vi "Main.vi"(0 "This Module":T1, 11 "error in (no error)":errorcluster) -> (15 "error out":errorcluster)   [LabVIEW 2017, in "Template.lvlib"]
doc: "This VI is the Module VI containing all the code required from this Module"
uses:
  Template.lvlib
  Modules.ctl
  Controls/Module - Data.ctl
  Controls/Module - States.ctl
  Controls/Timing - Data.ctl
  Controls/Process - Element.ctl
  Controls/Process.ctl
  Controls/Process - Status.ctl
  Controls/Timing - Mode.ctl
  Controls/Message - Queue Manager Mode.ctl
  Error Handler - Logger Module/Controls/Message.ctl
  Error Handler - Logger Module/Controls/Module - States.ctl
  Controls/FP - Update Value.ctl
  Controls/FP - Actionable Element.ctl
  Controls/FP - Enable_Disable.ctl
  Controls/Timing - Setup.ctl
  Error Handler - Logger Module/Error Handler - Logger.lvlib
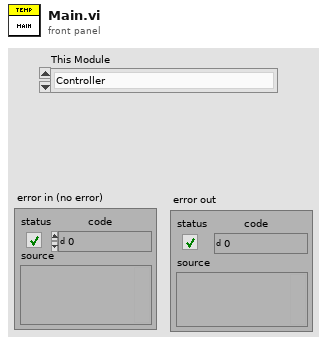
[diagram p1: front panel]
types:
  T1 = typedef "Error Handler - Logger.lvlib/Modules.ctl" = enum16{"Controller", "Error Handler - Logger"}
  T2 = typedef "Template.lvlib/Message - Queue Manager Mode.ctl" = enum16{"Create", "Get", "Destroy"}
  T3 = typedef "Template.lvlib/Timing - Mode.ctl" = enum16{"Reset", "Read", "Pause", "Resume"}
  T4 = typedef "Template.lvlib/Module - Data.ctl" = cluster{"This Module":T1, "Current State":T5, "Timing Data":T6, "Processes":T7[], "Log":string}
  T5 = typedef "Template.lvlib/Module - States.ctl" = enum16{"Initialize", "Event ", "Send data", "FP Element: Update", "FP Element: Disable/Enable", "Timer: Setup", "Terminate", "---------------Template---------------"}
  T6 = typedef "Template.lvlib/Timing - Data.ctl" = cluster{"Elapsed Time":dbl, "Time Target":dbl, "Time Stamp":timestamp, "Paused?":bool, "Reached?":bool}
  T7 = typedef "Template.lvlib/Process - Element.ctl" = cluster{"Process":T8, "Status":T9, "Data":variant}
  T8 = typedef "Template.lvlib/Process.ctl" = enum16{""}
  T9 = typedef "Template.lvlib/Process - Status.ctl" = enum16{"Uninitialized", "Busy"}
  T10 = typedef "Error Handler - Logger.lvlib/Message.ctl" = cluster{"State":T11, "Data":variant, "Originating Module":T1}
  T11 = typedef "Error Handler - Logger.lvlib/Module - States.ctl" = enum16{"Initialize", "Event ", "Send data", "FP Element: Update", "FP Element: Disable/Enable", "Timer: Setup", "Terminate", "--------Template----------", "Process Error", "Log ", "Log Error"}
  T12 = typedef "Template.lvlib/FP - Update Value.ctl" = cluster{"FP Element":T13, "Value":string}
  T13 = typedef "Template.lvlib/FP - Actionable Element.ctl" = enum16{"Put here all controls and indicators", "belonging to the UI of this module", "whose value can ", "be updated programatically", "or which can be enabled or disabled", ""}
  T14 = typedef "Template.lvlib/FP - Enable_Disable.ctl" = cluster{"FP Element":T13, "Enable?":bool}
  T15 = typedef "Template.lvlib/Timing - Setup.ctl" = cluster{"Mode":T3, "Update Time Target?":bool, "Time Target":dbl}
  T16 = typedef "Template.lvlib/Message.ctl" = cluster{"State":T5, "Data":variant, "Transitioning State?":bool}
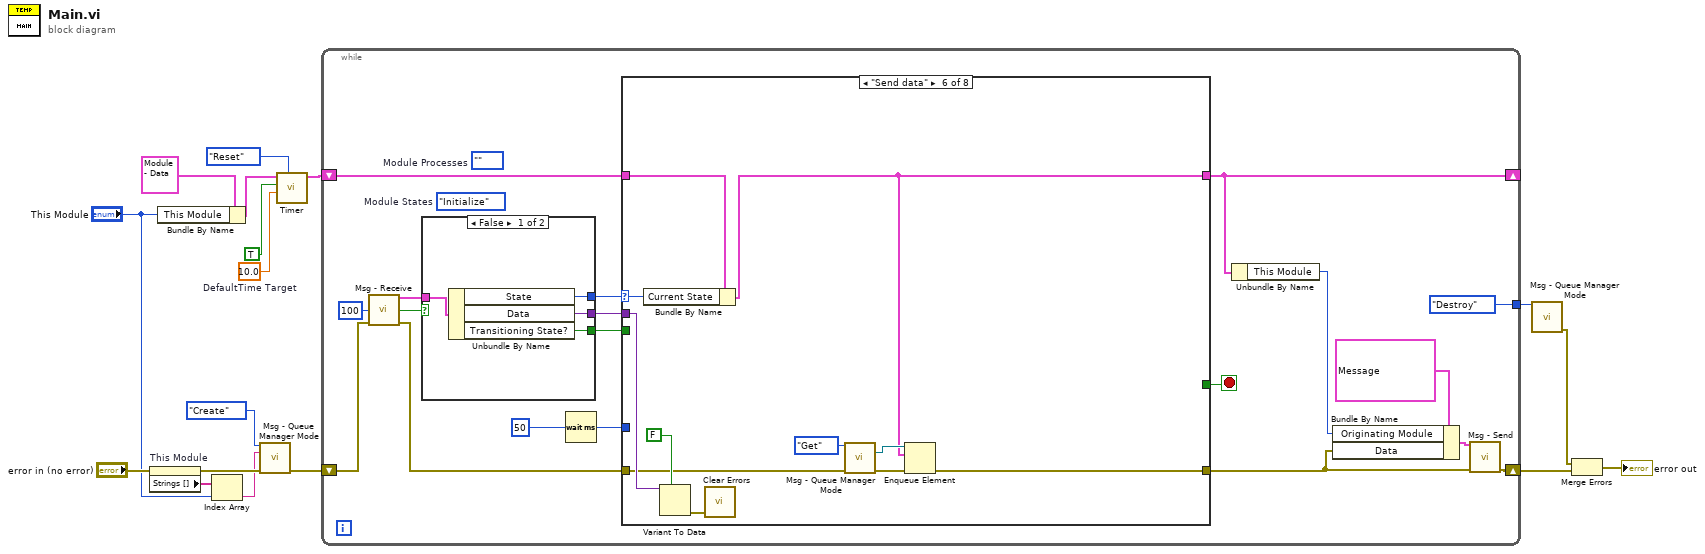
[diagram p0: block diagram]
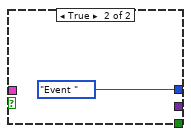
[diagram p2: hidden frame]
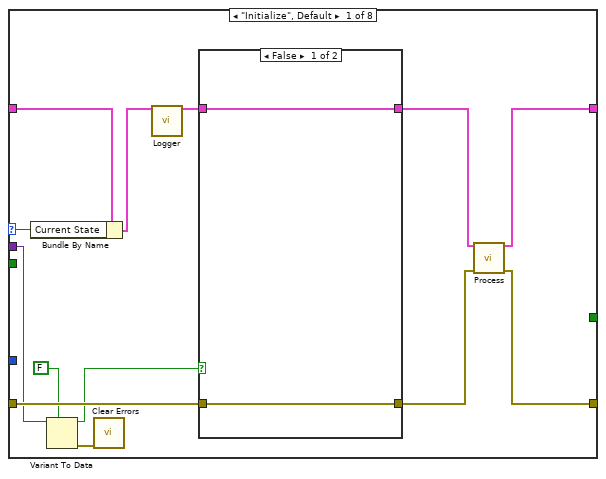
[diagram p3: hidden frame]
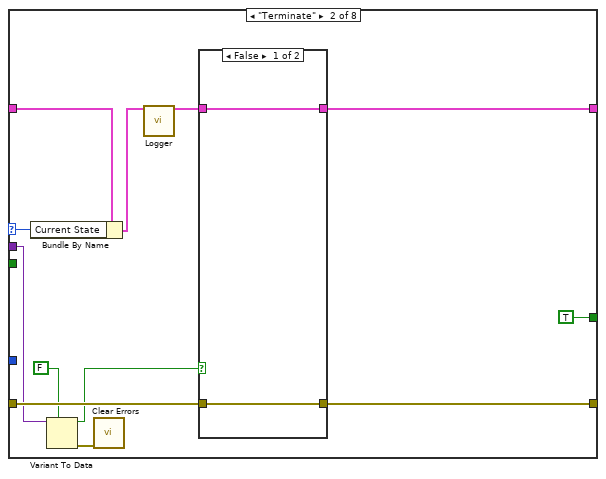
[diagram p5: hidden frame]
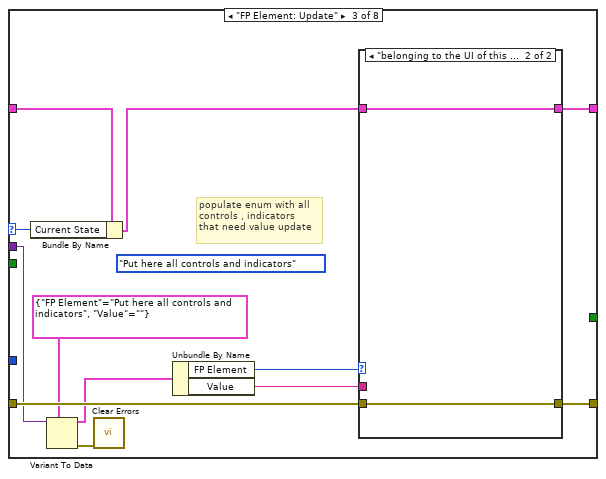
[diagram p7: hidden frame]
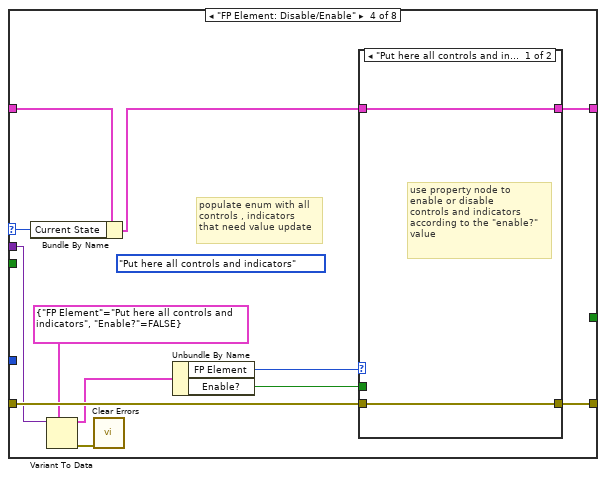
[diagram p9: hidden frame]
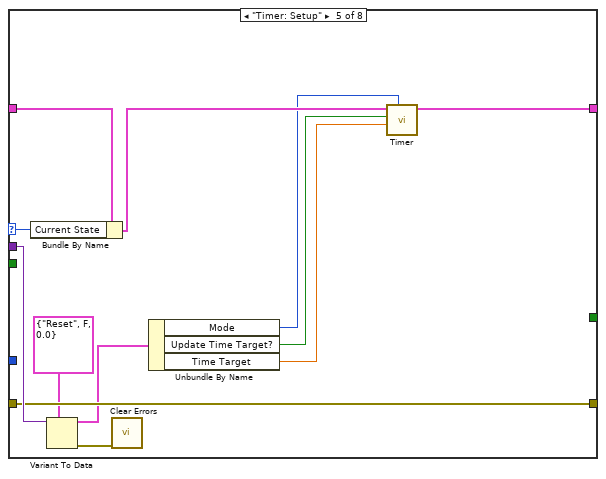
[diagram p11: hidden frame]
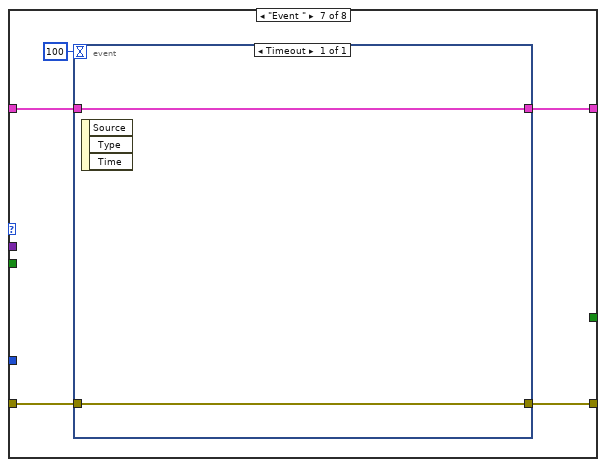
[diagram p12: hidden frame]
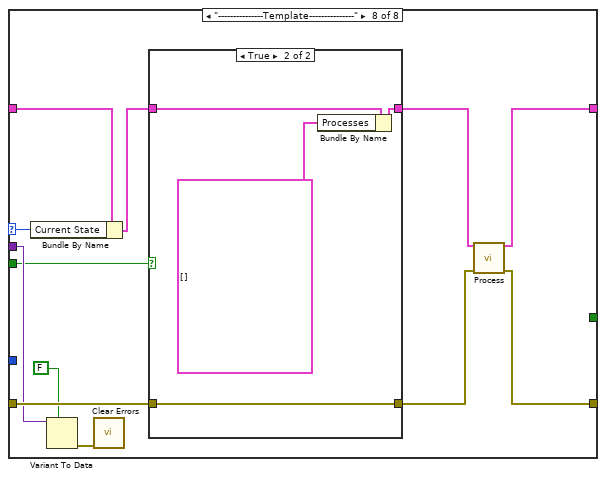
[diagram p13: hidden frame]
diagram:
  w13 = 10.0  # DefaultTime Target
  n1 = property on="This Module" class="Enum (strict)"(error in="error in (no error)") -> (error out=w8:errorcluster, "Strings []"=w10:string[])  [unwired: 1 in, 1 out]
  n2 = Bundle By Name(cluster=T4 {"This Module"=enum."Controller", "Current State"=enum."Initialize", "Timing Data"={"Elapsed Time"=0.0, "Time Target"=0.0, "Time Stamp"=timestamp(0 s since 1904-01-01), "Paused?"=FALSE, "Reached?"=FALSE}, "Processes"=[], "Log"=""} ("Module Data In"), "This Module"="This Module") -> (w16:T4)
  n3 = Index Array(array=w10, index="This Module") -> (element=w7:string)
  n4 = call "Msg - Queue Manager Mode.vi"("Mode"=Message_-_Queue_Manager_Mode."Create", "Module Name"=w7, "error in (no error)"=w8) -> ("error out"=w6:errorcluster)  [unwired: 10 in, 2 out]
  n5 = call "Timer.vi"("Mode"=Timing_-_Mode."Reset", "Time Target"=w13, "Update Target?"=TRUE, "Module Data In"=w16) -> ("Module Data Out"=w15:T4)  [unwired: 4 in, 3 out]
  n6 = while {
    shift-right: [w24] -> _
    shift-left: w15 -> [w36]
    shift-right: [w23] -> w3
    shift-left: w6 -> [w34]
    tunnel: [Message_-_Queue_Manager_Mode."Destroy" ("Mode")] -> w1
    stop <- w25 stop-if-true
    (unwired) Process.""  # Module Processes
    (unwired) Module_-_States."Initialize"  # Module States
    n7 = call "Msg - Receive.vi"("Timeout (ms)"=100, "error in (no error)"=w34) -> ("Message"=w30:T16, "timed out?"=w31:bool, "error out"=w33:errorcluster)  [unwired: 11 in]
    n8 = case shown="False" w31 {
      tunnel: w30 -> [w40 _]
      tunnel: [w39 Module_-_States."Event " ("State")] -> w29
      tunnel: [w38 _] -> w28
      tunnel: [w37 _] -> w19
      frame False {
        n9 = Unbundle By Name(w40) -> ("State"=w39:T5, "Data"=w38:variant, "Transitioning State?"=w37:bool)
      }
      frame True {
      }
    }
    n10 = Wait (ms)(milliseconds to wait=u32 50) -> (millisecond timer value=w26:u32)
    n11 = case shown="\"Send data\"" w29 {
      selector: w29 -> [w54 w70 w86 w102 w118 w129 _ w148]
      tunnel: [w48 w64 w81 w97 w110 w124 w131 w142] -> w24
      tunnel: w36 -> [w53 w69 w85 w101 w117 w128 w132 w147]
      tunnel: [w45 w63 w80 w96 w115 w122 w133 w139] -> w18
      tunnel: w33 -> [w52 w68 w83 w99 w115 w123 w134 w145]
      tunnel: w28 -> [w51 w67 w82 w98 w116 w127 _ w144]
      tunnel: w26 -> [_ _ _ _ _ _ _ _]
      tunnel: [_ TRUE _ _ _ _ _ _] -> w25
      tunnel: w19 -> [_ _ _ _ _ _ _ w137]
      frame "Initialize", Default {
        n12 = Bundle By Name(cluster=w53, "Current State"=w54) -> (w43:T4)
        n13 = Variant To Data(type=FALSE, Variant=w51) -> (data=w49:bool, error out=w44:errorcluster)  [unwired: 1 in]
        n14 = call <vilib>:"Clear Errors.vi"("error in (no error)"=w44) -> ()  [unwired: 5 in, 2 out]
        n15 = call "Logger.vi"("Module Data In"=w43) -> ("Module Data Out"=w42:T4)  [unwired: 13 in, 1 out]
        n16 = case shown="False" w49 {
          tunnel: w42 -> [w56 w58]
          tunnel: [w56 w58] -> w47
          tunnel: w52 -> [w55 w57]
          tunnel: [w55 w57] -> w46
          frame False {
          }
          frame True {
          }
        }
        n17 = call "Process.vi"("Module Data In"=w47, "error in (no error)"=w46) -> ("Module Data Out"=w48:T4, "error out"=w45:errorcluster)  [unwired: 12 in]
      }
      frame "Terminate" {
        n18 = Bundle By Name(cluster=w69, "Current State"=w70) -> (w60:T4)
        n19 = Variant To Data(type=FALSE, Variant=w67) -> (data=w65:bool, error out=w62:errorcluster)  [unwired: 1 in]
        n20 = call <vilib>:"Clear Errors.vi"("error in (no error)"=w62) -> ()  [unwired: 5 in, 2 out]
        n21 = call "Logger.vi"("Module Data In"=w60) -> ("Module Data Out"=w59:T4)  [unwired: 13 in, 1 out]
        n22 = case shown="False" w65 {
          tunnel: w59 -> [w72 w74]
          tunnel: [w72 w74] -> w64
          tunnel: w68 -> [w71 w73]
          tunnel: [w71 w73] -> w63
          frame False {
          }
          frame True {
          }
        }
      }
      frame "FP Element: Update" {
        (unwired) FP_-_Actionable_Element."Put here all controls and indicators" ("FP Element")
        # "populate enum with all\ncontrols , indicators \nthat need value update"
        n23 = Bundle By Name(cluster=w85, "Current State"=w86) -> (w84:T4)
        n24 = Variant To Data(type=T12 {"FP Element"=enum."Put here all controls and indicators", "Value"=""} ("Message"), Variant=w82) -> (data=w77:T12, error out=w79:errorcluster)  [unwired: 1 in]
        n25 = call <vilib>:"Clear Errors.vi"("error in (no error)"=w79) -> ()  [unwired: 5 in, 2 out]
        n26 = Unbundle By Name(w77) -> ("FP Element"=w76:T13, "Value"=w75:string)
        n27 = case shown="\"belonging to the UI of this module\"" w76 {
          tunnel: w84 -> [w88 w90]
          tunnel: [w88 w90] -> w81
          tunnel: w83 -> [w87 w89]
          tunnel: [w87 w89] -> w80
          tunnel: w75 -> [_ _]
          frame "Put here all controls and indicators", Default {
            # "use property node to\nupdate the values of\ncorresponding\ncontrols and indicators"
          }
          frame "belonging to the UI of this module" {
          }
        }
      }
      frame "FP Element: Disable/Enable" {
        (unwired) FP_-_Actionable_Element."Put here all controls and indicators" ("FP Element")
        # "populate enum with all\ncontrols , indicators \nthat need value update"
        n28 = Bundle By Name(cluster=w101, "Current State"=w102) -> (w100:T4)
        n29 = Variant To Data(type=T14 {"FP Element"=enum."Put here all controls and indicators", "Enable?"=FALSE} ("Message"), Variant=w98) -> (data=w94:T14, error out=w95:errorcluster)  [unwired: 1 in]
        n30 = call <vilib>:"Clear Errors.vi"("error in (no error)"=w95) -> ()  [unwired: 5 in, 2 out]
        n31 = Unbundle By Name(w94) -> ("FP Element"=w93:T13, "Enable?"=w92:bool)
        n32 = case shown="\"Put here all controls and indicators\", Default" w93 {
          tunnel: w100 -> [w104 w106]
          tunnel: [w104 w106] -> w97
          tunnel: w99 -> [w103 w105]
          tunnel: [w103 w105] -> w96
          tunnel: w92 -> [_ _]
          frame "Put here all controls and indicators", Default {
            # "use property node to\nenable or disable\ncontrols and indicators\naccording to the \"enable?\"\nvalue"
          }
          frame "belonging to the UI of this module" {
          }
        }
      }
      frame "Timer: Setup" {
        n33 = Bundle By Name(cluster=w117, "Current State"=w118) -> (w111:T4)
        n34 = Variant To Data(type=T15 {"Mode"=enum."Reset", "Update Time Target?"=FALSE, "Time Target"=0.0} ("Message"), Variant=w116) -> (data=w113:T15, error out=w114:errorcluster)  [unwired: 1 in]
        n35 = call <vilib>:"Clear Errors.vi"("error in (no error)"=w114) -> ()  [unwired: 5 in, 2 out]
        n36 = Unbundle By Name(w113) -> ("Mode"=w109:T3, "Update Time Target?"=w108:bool, "Time Target"=w107:dbl)
        n37 = call "Timer.vi"("Mode"=w109, "Time Target"=w107, "Update Target?"=w108, "Module Data In"=w111) -> ("Module Data Out"=w110:T4)  [unwired: 4 in, 3 out]
      }
      frame "Send data" {
        n38 = Bundle By Name(cluster=w128, "Current State"=w129) -> (w124:T4)
        n39 = Variant To Data(type=FALSE, Variant=w127) -> (error out=w120:errorcluster)  [unwired: 1 in, 1 out]
        n40 = call <vilib>:"Clear Errors.vi"("error in (no error)"=w120) -> ()  [unwired: 5 in, 2 out]
        n41 = call "Msg - Queue Manager Mode.vi"("Mode"=Message_-_Queue_Manager_Mode."Get", "error in (no error)"=w123) -> (">>Controller"=w125:refnum<queue>, "error out"=w121:errorcluster)  [unwired: 11 in, 1 out]
        n42 = Enqueue Element(queue=w125, element=w124, error in (no error)=w121) -> (error out=w122:errorcluster)  [unwired: 1 in, 2 out]
      }
      frame "Event " {
        n43 = event shown="[0] Timeout" {
          selector: _ -> [_]
          dyn-events: _ -> [_]
          timeout: 100 -> [_]
          tunnel: w134 -> [w136]
          tunnel: [w136] -> w133
          tunnel: w132 -> [w135]
          tunnel: [w135] -> w131
          event Timeout {
            n44 = event-data() -> ()  [unwired: 1 in, 3 out]
          }
        }
      }
      frame "---------------Template---------------" {
        n45 = Bundle By Name(cluster=w147, "Current State"=w148) -> (w146:T4)
        n46 = Variant To Data(type=FALSE, Variant=w144) -> (error out=w138:errorcluster)  [unwired: 1 in, 1 out]
        n47 = call <vilib>:"Clear Errors.vi"("error in (no error)"=w138) -> ()  [unwired: 5 in, 2 out]
        n48 = case shown="True" w137 {
          tunnel: w146 -> [w150 w152]
          tunnel: [w150 w151] -> w141
          tunnel: w145 -> [w149 w154]
          tunnel: [w149 w154] -> w140
          frame False {
          }
          frame True {
            n49 = Bundle By Name(cluster=w152, "Processes"=T7[] []) -> (w151:T4)
          }
        }
        n50 = call "Process.vi"("Module Data In"=w141, "error in (no error)"=w140) -> ("Module Data Out"=w142:T4, "error out"=w139:errorcluster)  [unwired: 12 in]
      }
    }
    n51 = Unbundle By Name(w24) -> ("This Module"=w20:T1)
    n52 = Bundle By Name(cluster=T10 {"State"=enum."Process Error", "Data"=variant, "Originating Module"=enum."Controller"} ("Message"), "Originating Module"=w20, "Data"=w18) -> (w21:T10)
    n53 = call "Msg - Send.vi"("Message"=w21, "error in (no error)"=w18) -> ("error out"=w23:errorcluster)  [unwired: 13 in]
  }
  n54 = call "Msg - Queue Manager Mode.vi"("Mode"=w1) -> ("error out"=w4:errorcluster)  [unwired: 12 in, 2 out]
  n55 = Merge Errors(w4, w3) -> (→"error out":errorcluster)
